vi "ZMC Make Zar.vi"(7 "uid":u32, 8 "error in (no error)":errorcluster caption="错误输入（无错误）", 9 "pPass":string, 10 "pZarfilename":string, 11 "pZpjfilename":string) -> (0 "error out":errorcluster caption="错误输出", 3 "function return":i32)   [LabVIEW 2015, in "zauxdll.lvlib"]
doc: "int32 __stdcall ZMC_MakeZar(const char* pZpjfilename, const char* pZarfilename, const char *pPass, uint32 uid);"
uses:
  zauxdll.lvlib
  zmotion.dll
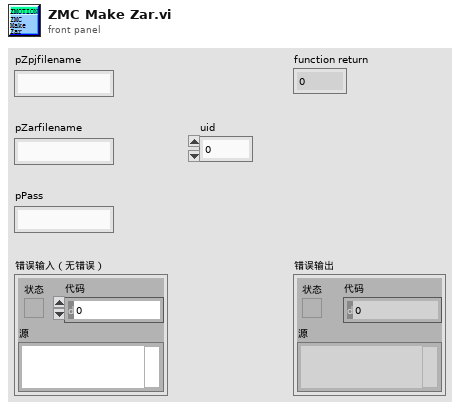
[diagram p1: front panel]
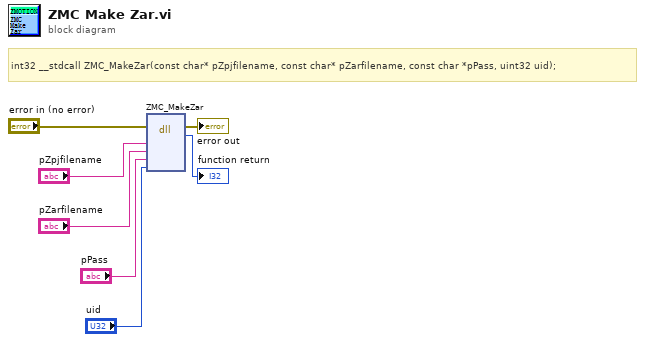
[diagram p0: block diagram]
diagram:
  # "int32 __stdcall ZMC_MakeZar(const char* pZpjfilename, const char* pZarfilename, const char *pPass, uint32 uid);"
  n1 = dll-call lib="C:/Users/VIC/Desktop/GOGORO_SA/system/LLB/zmotion/zaux/zmotion.*" fn="ZMC_MakeZar"(error in="error in (no error)", "pZpjfilename"="pZpjfilename", "pZarfilename"="pZarfilename", "pPass"="pPass", "uid"="uid") -> (error out=→"error out":errorcluster, →"function return":i32)  [unwired: 6 in, 1 out]
